vi "Fill FN - Initial Mass (SubVI).vi"(0 "Signals IN":T1={"Dispense"=FALSE, "Fill"=FALSE, "Spray"=FALSE, "Drain"=TRUE, "Complete"=FALSE, "Fill Error"=FALSE, "Disp. Error"=FALSE, "Fill Timeout"=FALSE, "Disp. Timeout"=FALSE, "Purge"=TRUE}, 2 "Measured Mass (g)":dbl(knob) scale=0.0..1000.0, 3 "Main Case Change?":bool) -> (14 "Signals OUT":T1={"Dispense"=FALSE, "Fill"=FALSE, "Spray"=FALSE, "Drain"=TRUE, "Complete"=FALSE, "Fill Error"=FALSE, "Disp. Error"=FALSE, "Fill Timeout"=FALSE, "Disp. Timeout"=FALSE, "Purge"=TRUE}, 16 "Initial Mass":dbl, 17 "Fill Error":bool, 19 "Case Complete":bool)   [LabVIEW 2011]
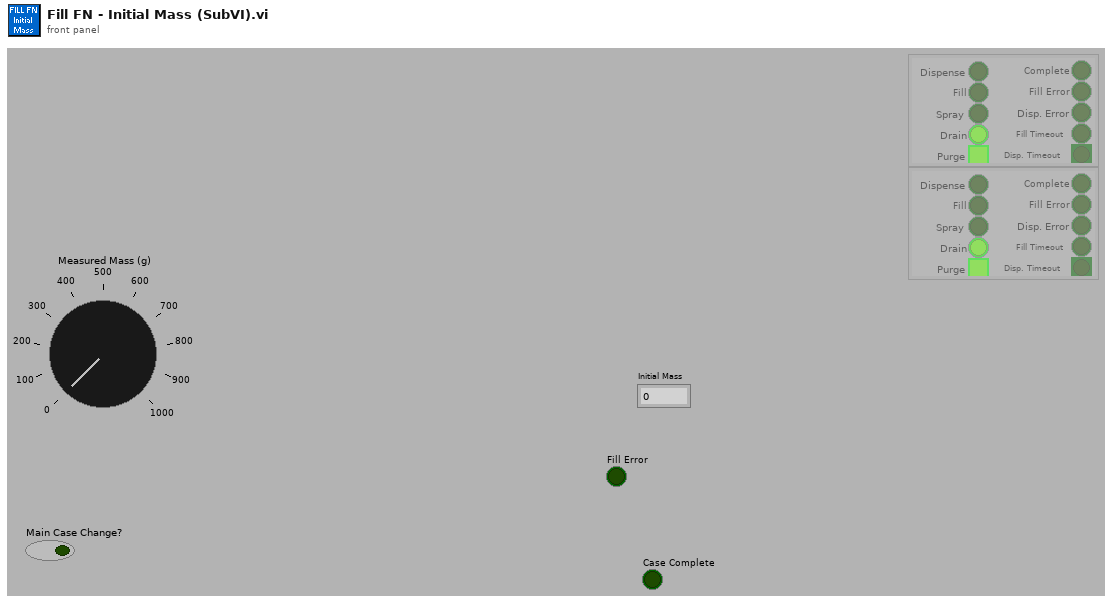
[diagram p1: front panel]
types:
  T1 = cluster{"Dispense":bool, "Fill":bool, "Spray":bool, "Drain":bool, "Complete":bool, "Fill Error":bool, "Disp. Error":bool, "Fill Timeout":bool, "Disp. Timeout":bool, "Purge":bool}
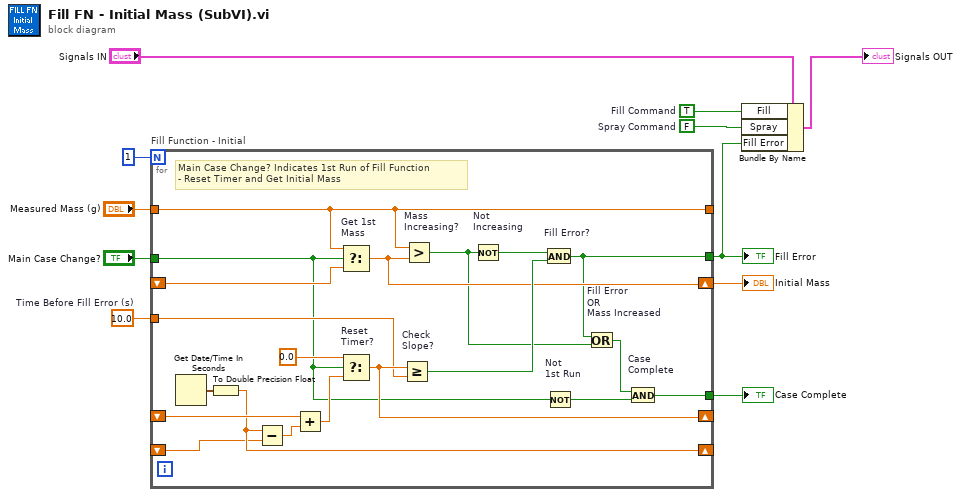
[diagram p0: block diagram]
diagram:
  w3 = FALSE  # Spray Command
  w4 = TRUE  # Fill Command
  w9 = 10.0  # Time Before Fill Error (s)
  n1 = for "Fill Function - Initial" {
    N: 1 -> [_]
    shift-right: [w23] -> _
    shift-left: _ -> [w31]
    shift-right: [w28] -> _
    shift-left: _ -> [w27]
    tunnel: "Measured Mass (g)" -> [w18]
    tunnel: "Main Case Change?" -> [w14]
    shift-right: [w19] -> w6
    shift-left: _ -> [w22]
    tunnel: w9 -> [w20]
    tunnel: [w17] -> w5
    tunnel: [w18] -> _
    tunnel: [w13] -> w7
    # "Main Case Change? Indicates 1st Run of Fill Function\n- Reset Timer and Get Initial Mass"
    n2 = Get Date/Time In Seconds() -> (seconds since 1Jan1904=w30:timestamp)
    n3 = To Double Precision Float(number=w30) -> (double precision float=w28:dbl)
    n4 = Subtract(x=w28, y=w27) -> (x-y=w26:dbl)
    n5 = Add(x=w31, y=w26) -> (x+y=w29:dbl)
    n6 = Select "Get 1st\nMass"(t=w18, s=w14, f=w22) -> (s? t:f=w19:dbl)
    n7 = Select "Reset\nTimer?"(t=0.0, s=w14, f=w29) -> (s? t:f=w23:dbl)
    n8 = Greater Or Equal? "Check\nSlope?"(x=w23, y=w20) -> (x >= y?=w24:bool)
    n9 = Greater? "Mass\nIncreasing?"(x=w18, y=w19) -> (0:w16:bool)
    n10 = Not "Not\nIncreasing"(x=w16) -> (.not. x?=w21:bool)
    n11 = And "Fill Error?"(x=w21, y=w24) -> (x .and. y?=w17:bool)
    n12 = Not "Not\n1st Run"(x=w14) -> (.not. x?=w12:bool)
    n13 = Or "Fill Error\nOR\nMass Increased"(x=w17, y=w16) -> (x .or. y?=w15:bool)
    n14 = And "Case\nComplete"(x=w15, y=w12) -> (x .and. y?=w13:bool)
  }
  "Fill Error" <- w5
  "Case Complete" <- w7
  "Initial Mass" <- w6
  n15 = Bundle By Name(cluster="Signals IN", "Fill"=w4, "Spray"=w3, "Fill Error"=w5) -> (→"Signals OUT":T1)
